vi "Example CaseStructure.vi"(8 "Error In":errorcluster) -> (0 "Error Out":errorcluster, 1 "signal out":waveform(dbl), 2 "signal out 2":waveform(dbl), 3 "appended array":waveform(dbl)[](array[waveform]))   [LabVIEW 2014]
uses:
  <vilib>/measure/NI_MABase.lvlib
panel:
  in  "Numeric":u8
  in  "Boolean":bool
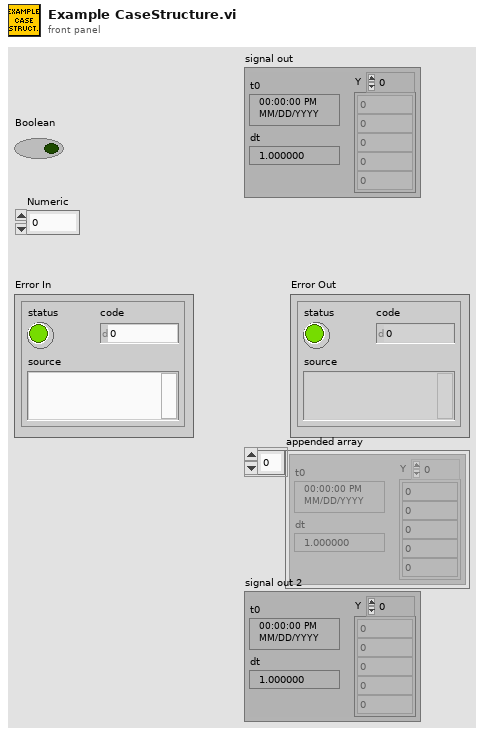
[diagram p1: front panel]
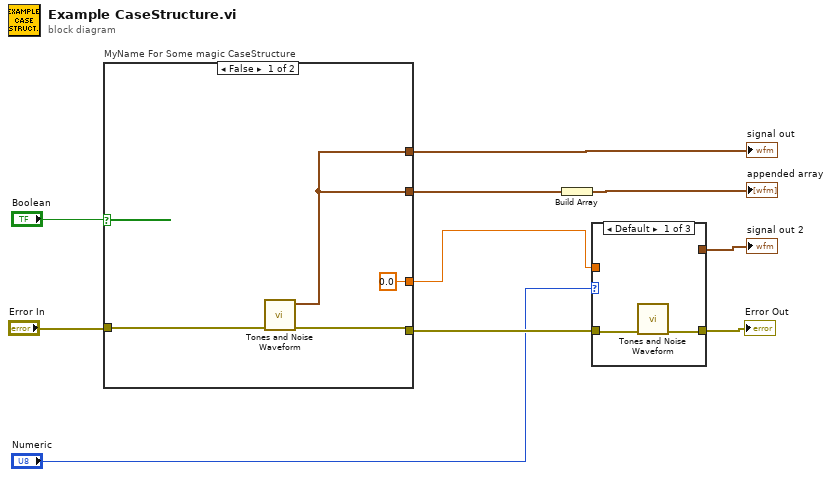
[diagram p0: block diagram]
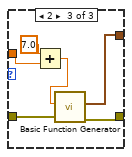
[diagram p3: hidden frame]
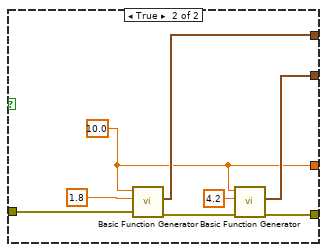
[diagram p4: hidden frame]
diagram:
  n1 = case "MyName For Some magic CaseStructure" shown="False" "Boolean" {
    tunnel: "Error In" -> [w14 w22]
    tunnel: [w13 w20] -> w4
    tunnel: [w12 w17] -> w8
    tunnel: [w12 w16] -> w7
    tunnel: [0.0 ("frequency") w15] -> w2
    frame False {
      n2 = call <vilib>:"Tones and Noise Waveform.vi"("error in (no error)"=w14) -> ("error out"=w13:errorcluster, "signal out"=w12:waveform(dbl))  [unwired: 9 in]
    }
    frame True {
      w15 = 10.0 ("frequency")
      n3 = call <vilib>:"Basic Function Generator.vi"("error in (no error)"=w22, "amplitude"=1.8, "frequency"=w15) -> ("error out"=w21:errorcluster, "signal out"=w17:waveform(dbl))  [unwired: 6 in, 1 out]
      n4 = call <vilib>:"Basic Function Generator.vi"("error in (no error)"=w21, "amplitude"=4.2, "frequency"=w15) -> ("error out"=w20:errorcluster, "signal out"=w16:waveform(dbl))  [unwired: 6 in, 1 out]
    }
  }
  "signal out" <- w8
  n5 = Build Array(w7) -> (→"appended array":waveform(dbl)[])
  n6 = case shown="Default" "Numeric" {
    tunnel: [w24 w25 w31] -> w5
    tunnel: w4 -> [w23 w25 w30]
    tunnel: w2 -> [_ _ w27]
    tunnel: [_ _ w26] -> w1
    frame Default {
      n7 = call <vilib>:"Tones and Noise Waveform.vi"("error in (no error)"=w23) -> ("error out"=w24:errorcluster)  [unwired: 9 in, 1 out]
    }
    frame 1 {
    }
    frame 2 {
      n8 = Add(x=7.0, y=w27) -> (x+y=w28:dbl)
      n9 = call <vilib>:"Basic Function Generator.vi"("error in (no error)"=w30, "amplitude"=w28) -> ("error out"=w31:errorcluster, "signal out"=w26:waveform(dbl))  [unwired: 7 in, 1 out]
    }
  }
  "Error Out" <- w5
  "signal out 2" <- w1
